vi "ManipIntake.vi"(1 "Time Since Latch":u32, 2 "Instruction String":string) -> (0 "Advance Trigger":bool)   [LabVIEW 2019]
uses:
  dsinstructions.vi
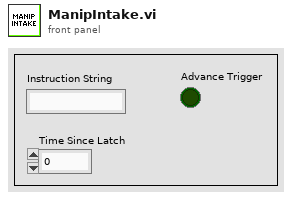
[diagram p1: front panel]
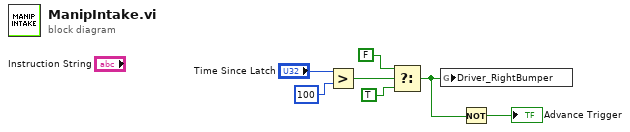
[diagram p0: block diagram]
diagram:
  n1 = Greater?(x="Time Since Latch", y=u32 100) -> (0:w5:bool)
  n2 = Select(t=FALSE, s=w5, f=TRUE ("Driver_RightBumper")) -> (s? t:f=w2:bool)
  n3 = global write "dsinstructions.vi" "Driver_RightBumper"(w2) -> ()
  n4 = Not(x=w2) -> (.not. x?=→"Advance Trigger":bool)
